vi "Sequence.SerialsFglb.vi"(7 "Action (get)":T6=enum."get", 8 "error in":errorcluster, 9 "Printed serials in":i32[](array[numeric]), 10 "Serial data in":T4, 11 "Counters in":T3) -> (0 "error out":errorcluster, 1 "Printed serials out":i32[](array[numeric]), 2 "Serial out":i32, 3 "Counters out":T3, 5 "StatusFlags":T2)   [LabVIEW 2016]
uses:
  Sequence.SerialsFglb.Action.ctl
  Sequence.SerialsFglb.SerialData.ctl
  Station/Station.ProductSlot.ctl
  Sequence.Counters.ctl
  Sequence.SerialsFglb.StatusFlags.ctl
  Sequence.SerialsFglb.Data.ctl
  Global/ApplicationGlobal.vi
panel:
  out "Serials":T1[](array[typedef])
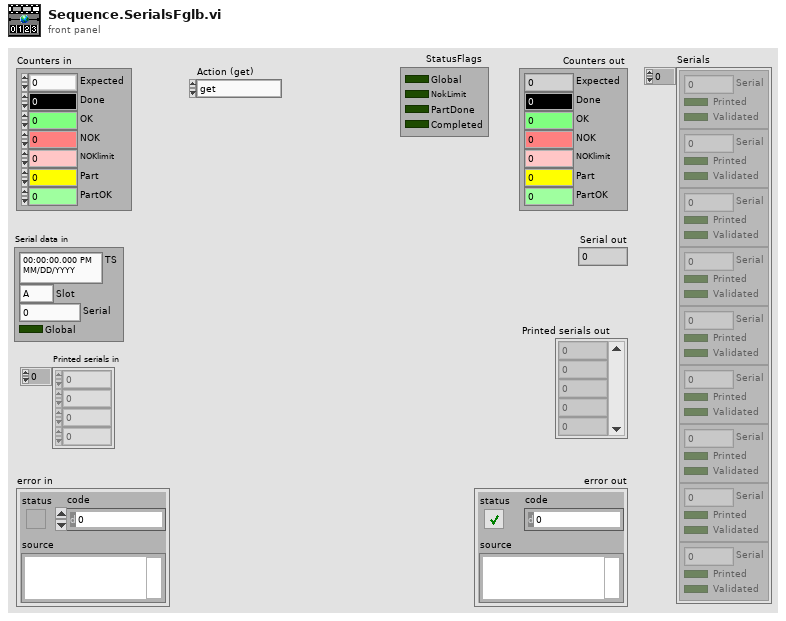
[diagram p1: front panel]
types:
  T1 = typedef "Sequence.SerialsFglb.Data.ctl" = cluster{"Serial":i32, "Printed":bool, "Validated":bool}
  T2 = typedef "Sequence.SerialsFglb.StatusFlags.ctl" = cluster{"Global":bool, "NokLimit":bool, "PartDone":bool, "Completed":bool}
  T3 = typedef "Sequence.Counters.ctl" = cluster{"Expected":u16, "Done":u16, "OK":u16, "NOK":u16, "NOKlimit":u16, "Part":u16, "PartOK":u16}
  T4 = typedef "Sequence.SerialsFglb.SerialData.ctl" = cluster{"TS":timestamp, "Slot":T5, "Serial":i32, "Global":bool}
  T5 = typedef "Station.ProductSlot.ctl" = enum8{"A", "B"}
  T6 = typedef "Sequence.SerialsFglb.Action.ctl" = enum16{"init", "get", "get next", "pass", "fail", "confirm", "clean"}
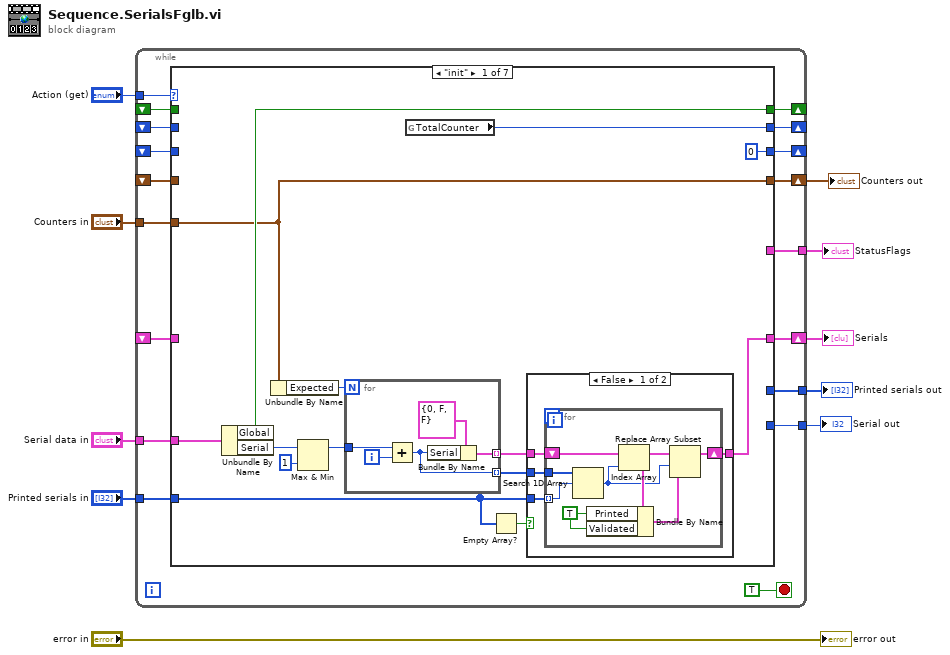
[diagram p0: block diagram]
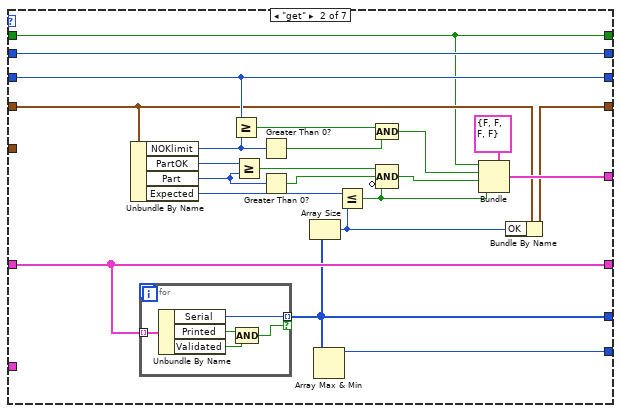
[diagram p3: hidden frame]
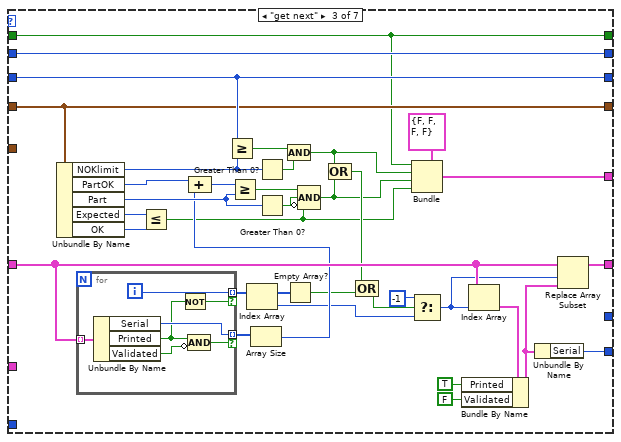
[diagram p4: hidden frame]
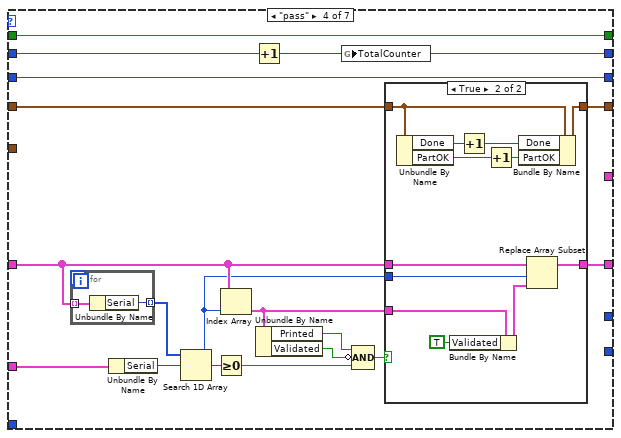
[diagram p5: hidden frame]
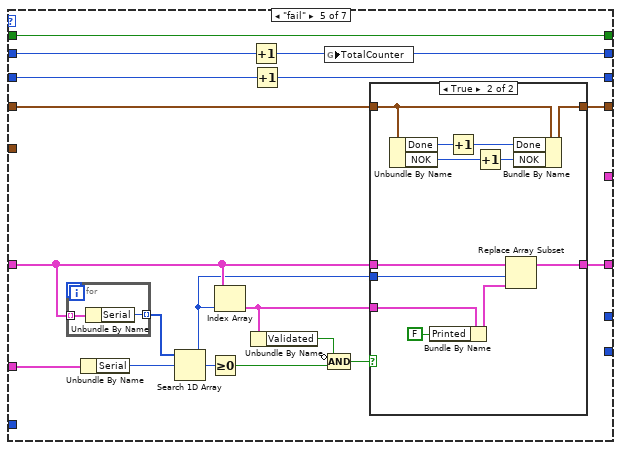
[diagram p7: hidden frame]
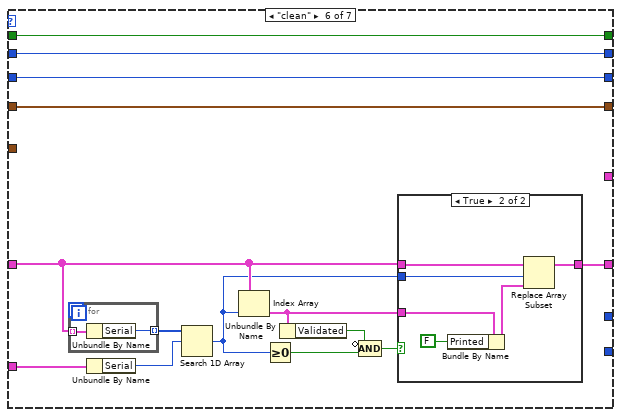
[diagram p9: hidden frame]
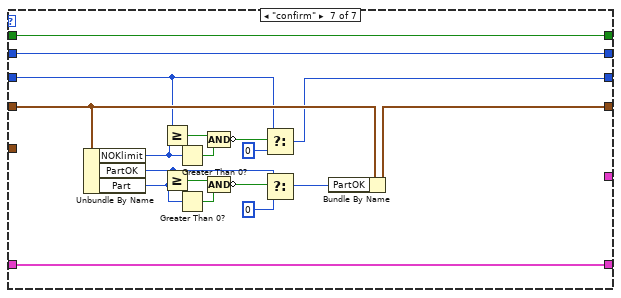
[diagram p11: hidden frame]
diagram:
  n1 = while {
    tunnel: "Action (get)" -> [w27]
    shift-right: [w26] -> w1
    shift-left: _ -> [w25]
    tunnel: [w24] -> w8
    tunnel: "Serial data in" -> [w23]
    tunnel: "Printed serials in" -> [w22]
    tunnel: [w21] -> w5
    shift-right: [w20] -> _
    shift-left: _ -> [w19]
    shift-right: [w17] -> w3
    shift-left: _ -> [w18]
    tunnel: "Counters in" -> [w16]
    shift-right: [w15] -> _
    shift-left: _ -> [w14]
    shift-right: [w13] -> _
    shift-left: _ -> [w12]
    tunnel: [w11] -> w2
    stop <- TRUE stop-if-true
    n2 = case shown="\"init\"" w27 {
      tunnel: [w34 w82 w122 w136 w179 w209 w221] -> w26
      tunnel: w25 -> [_ w82 w121 w137 w169 w208 w221]
      tunnel: [_ w81 w88 _ _ _ _] -> w24
      tunnel: w23 -> [w42 _ _ w145 w165 w207 _]
      tunnel: w22 -> [w37 _ _ _ _ _ _]
      tunnel: [_ w68 _ _ _ _ _] -> w21
      tunnel: [w33 w66 w97 w144 w178 w206 w220] -> w20
      tunnel: w19 -> [_ w66 w97 w144 w178 w206 w220]
      tunnel: w18 -> [_ w70 w106 w140 w174 w203 w226]
      tunnel: [w32 w69 w106 w143 w173 w203 w225] -> w17
      tunnel: w16 -> [w32 _ _ _ _ _ _]
      tunnel: [w29 w80 w117 w139 w172 w205 w222] -> w15
      tunnel: w14 -> [_ w80 w117 w142 w177 w205 w222]
      tunnel: [0 w74 w111 w141 w176 w204 w219] -> w13
      tunnel: w12 -> [_ w74 w111 w141 w175 w204 w223]
      tunnel: [_ w71 w108 _ _ _ _] -> w11
      frame "init" {
        n3 = Unbundle By Name(w42) -> ("Global"=w33:bool, "Serial"=w41:i32)
        n4 = Unbundle By Name(w32) -> ("Expected"=w31:u16)
        n5 = Max & Min(x=w41, y=1) -> (max(x,y)=w35:i32)  [unwired: 1 out]
        n6 = for {
          N: w31 -> [_]
          tunnel: w35 -> [w60]
          tunnel: [w57] -> w39 mode=indexing
          tunnel: [w56] -> w38 mode=indexing
          i -> [w59]
          n7 = Add(x=w60, y=w59) -> (x+y=w56:i32)
          n8 = Bundle By Name(cluster=T1 {"Serial"=0, "Printed"=FALSE, "Validated"=FALSE} ("Data"), "Serial"=w56) -> (w57:T1)
        }
        n9 = global read "ApplicationGlobal.vi" "TotalCounter"() -> (w29:u32)
        n10 = Empty Array?(array=w37) -> (empty?=w36:bool)
        n11 = case shown="False" w36 {
          tunnel: w39 -> [w46 w55]
          tunnel: w38 -> [w45 _]
          tunnel: w37 -> [w44 _]
          tunnel: [w43 w55] -> w34
          frame False {
            n12 = for {
              tunnel: w45 -> [w54]
              tunnel: w44 -> [w53] mode=indexing
              shift-right: [w52] -> w43
              shift-left: w46 -> [w51]
              w49 = TRUE ("Printed")
              n13 = Search 1D Array(1D array=w54, element=w53) -> (index of element=w47:i32)  [unwired: 1 in]
              n14 = Index Array(array=w51, index=w47) -> (element=w50:T1)
              n15 = Bundle By Name(cluster=w50, "Printed"=w49, "Validated"=w49) -> (w48:T1)
              n16 = Replace Array Subset(array=w51, new element=w48, index=w47) -> (w52:T1[])
            }
          }
          frame True {
          }
        }
      }
      frame "get" {
        n17 = Unbundle By Name(w70) -> ("NOKlimit"=w73:u16, "PartOK"=w75:u16, "Part"=w76:u16, "Expected"=w67:u16)
        n18 = for {
          tunnel: w82 -> [w87] mode=indexing
          tunnel: [w86] -> w68 mode=indexing if=w83
          n19 = Unbundle By Name(w87) -> ("Serial"=w86:i32, "Printed"=w85:bool, "Validated"=w84:bool)
          n20 = Compound Arithmetic op=AND(w85, w84) -> (w83:bool)
        }
        n21 = Greater Or Equal?(x=w74, y=w73) -> (x >= y?=w79:bool)
        n22 = Greater Or Equal?(x=w75, y=w76) -> (x >= y?=w77:bool)
        n23 = Greater Than 0?(x=w73) -> (x > 0?=w78:bool)
        n24 = Greater Than 0?(x=w76) -> (x > 0?=w62:bool)
        n25 = Array Size(array=w68) -> (size(s)=w63:i32)
        n26 = Array Max & Min(array=w68) -> (max value=w81:i32)  [unwired: 3 out]
        n27 = Less Or Equal?(x=w67, y=w63) -> (x <= y?=w61:bool)
        n28 = Compound Arithmetic op=AND(w79, w78) -> (w65:bool)
        n29 = Compound Arithmetic op=AND(w77, w62, invert w61) -> (w64:bool)
        n30 = Bundle(cluster=T2 {"Global"=FALSE, "NokLimit"=FALSE, "PartDone"=FALSE, "Completed"=FALSE} ("StatusFlags"), "Global"=w66, "NokLimit"=w65, "PartDone"=w64, "Completed"=w61) -> (w71:T2)
        n31 = Bundle By Name(cluster=w70, "OK"=w63) -> (w69:T3)
      }
      frame "get next" {
        n32 = Unbundle By Name(w106) -> ("NOKlimit"=w112:u16, "PartOK"=w104:u16, "Part"=w113:u16, "Expected"=w94:u16, "OK"=w93:u16)
        n33 = for {
          tunnel: w121 -> [w129] mode=indexing
          tunnel: [w128] -> w101 mode=indexing if=w127
          tunnel: [w126] -> w105 mode=indexing if=w124
          i -> [w128]
          n34 = Unbundle By Name(w129) -> ("Serial"=w126:i32, "Printed"=w125:bool, "Validated"=w123:bool)
          n35 = Not(x=w125) -> (.not. x?=w127:bool)
          n36 = Compound Arithmetic op=AND(w125, invert w123) -> (w124:bool)
        }
        n37 = Less Or Equal?(x=w94, y=w93) -> (x <= y?=w91:bool)
        n38 = Greater Or Equal?(x=w111, y=w112) -> (x >= y?=w116:bool)
        n39 = Index Array(array=w101) -> (element=w98:i32)  [unwired: 1 in]
        n40 = Array Size(array=w105) -> (size(s)=w102:i32)
        n41 = Compound Arithmetic op=ADD(w104, w102) -> (w103:i32)
        n42 = Greater Or Equal?(x=w103, y=w113) -> (x >= y?=w114:bool)
        n43 = Greater Than 0?(x=w112) -> (x > 0?=w115:bool)
        n44 = Greater Than 0?(x=w113) -> (x > 0?=w92:bool)
        n45 = Empty Array?(array=w101) -> (empty?=w100:bool)
        n46 = Compound Arithmetic op=AND(w116, w115) -> (w96:bool)
        n47 = Compound Arithmetic op=AND(w114, w92, invert w91) -> (w95:bool)
        n48 = Compound Arithmetic op=OR(w96, w95) -> (w110:bool)
        n49 = Compound Arithmetic op=OR(w110, w100) -> (w107:bool)
        n50 = Bundle(cluster=T2 {"Global"=FALSE, "NokLimit"=FALSE, "PartDone"=FALSE, "Completed"=FALSE} ("StatusFlags"), "Global"=w97, "NokLimit"=w96, "PartDone"=w95, "Completed"=w91) -> (w108:T2)
        n51 = Select(t=-1 ("f"), s=w107, f=w98) -> (s? t:f=w120:i32)
        n52 = Index Array(array=w121, index=w120) -> (element=w119:T1)
        n53 = Bundle By Name(cluster=w119, "Printed"=TRUE, "Validated"=FALSE) -> (w89:T1)
        n54 = Unbundle By Name(w89) -> ("Serial"=w88:i32)
        n55 = Replace Array Subset(array=w121, new element=w89, index=w120) -> (w122:T1[])
      }
      frame "pass" {
        n56 = for {
          tunnel: w137 -> [w148] mode=indexing
          tunnel: [w147] -> w146 mode=indexing
          n57 = Unbundle By Name(w148) -> ("Serial"=w147:i32)
        }
        n58 = Unbundle By Name(w145) -> ("Serial"=w132:i32)
        n59 = Search 1D Array(1D array=w146, element=w132) -> (index of element=w134:i32)  [unwired: 1 in]
        n60 = Greater Or Equal To 0?(x=w134) -> (x >= 0?=w133:bool)
        n61 = Index Array(array=w137, index=w134) -> (element=w135:T1)
        n62 = Increment(x=w142) -> (x+1=w139:u32)
        n63 = Unbundle By Name(w135) -> ("Printed"=w130:bool, "Validated"=w131:bool)
        n64 = global write "ApplicationGlobal.vi" "TotalCounter"(w139) -> ()
        n65 = Compound Arithmetic op=AND(w130, invert w131, w133) -> (w138:bool)
        n66 = case shown="True" w138 {
          tunnel: w140 -> [w150 w162]
          tunnel: [w150 w161] -> w143
          tunnel: w137 -> [w149 w156]
          tunnel: [w149 w155] -> w136
          tunnel: w135 -> [_ w154]
          tunnel: w134 -> [_ w153]
          frame False {
          }
          frame True {
            n67 = Unbundle By Name(w162) -> ("Done"=w152:u16, "PartOK"=w160:u16)
            n68 = Bundle By Name(cluster=w154, "Validated"=TRUE ("Printed")) -> (w158:T1)
            n69 = Increment(x=w152) -> (x+1=w151:u16)
            n70 = Increment(x=w160) -> (x+1=w159:u16)
            n71 = Bundle By Name(cluster=w162, "Done"=w151, "PartOK"=w159) -> (w161:T3)
            n72 = Replace Array Subset(array=w156, new element=w158, index=w153) -> (w155:T1[])
          }
        }
      }
      frame "fail" {
        n73 = for {
          tunnel: w169 -> [w195] mode=indexing
          tunnel: [w194] -> w171 mode=indexing
          n74 = Unbundle By Name(w195) -> ("Serial"=w194:i32)
        }
        n75 = Unbundle By Name(w165) -> ("Serial"=w164:i32)
        n76 = Search 1D Array(1D array=w171, element=w164) -> (index of element=w166:i32)  [unwired: 1 in]
        n77 = Greater Or Equal To 0?(x=w166) -> (x >= 0?=w170:bool)
        n78 = Index Array(array=w169, index=w166) -> (element=w168:T1)
        n79 = Increment(x=w177) -> (x+1=w172:u32)
        n80 = Unbundle By Name(w168) -> ("Validated"=w163:bool)
        n81 = Increment(x=w175) -> (x+1=w176:i32)
        n82 = global write "ApplicationGlobal.vi" "TotalCounter"(w172) -> ()
        n83 = Compound Arithmetic op=AND(invert w163, w170) -> (w167:bool)
        n84 = case shown="True" w167 {
          tunnel: [w180 w193] -> w179
          tunnel: w174 -> [w181 w189]
          tunnel: [w181 w186] -> w173
          tunnel: w169 -> [w180 w184]
          tunnel: w168 -> [_ w183]
          tunnel: w166 -> [_ w182]
          frame False {
          }
          frame True {
            n85 = Unbundle By Name(w189) -> ("Done"=w190:u16, "NOK"=w188:u16)
            n86 = Bundle By Name(cluster=w183, "Printed"=FALSE) -> (w192:T1)
            n87 = Increment(x=w190) -> (x+1=w191:u16)
            n88 = Increment(x=w188) -> (x+1=w187:u16)
            n89 = Replace Array Subset(array=w184, new element=w192, index=w182) -> (w193:T1[])
            n90 = Bundle By Name(cluster=w189, "Done"=w191, "NOK"=w187) -> (w186:T3)
          }
        }
      }
      frame "clean" {
        n91 = for {
          tunnel: w208 -> [w218] mode=indexing
          tunnel: [w217] -> w202 mode=indexing
          n92 = Unbundle By Name(w218) -> ("Serial"=w217:i32)
        }
        n93 = Unbundle By Name(w207) -> ("Serial"=w200:i32)
        n94 = Search 1D Array(1D array=w202, element=w200) -> (index of element=w201:i32)  [unwired: 1 in]
        n95 = Index Array(array=w208, index=w201) -> (element=w199:T1)
        n96 = Greater Or Equal To 0?(x=w201) -> (x >= 0?=w198:bool)
        n97 = Unbundle By Name(w199) -> ("Validated"=w196:bool)
        n98 = Compound Arithmetic op=AND(invert w196, w198) -> (w197:bool)
        n99 = case shown="True" w197 {
          tunnel: [w210 w216] -> w209
          tunnel: w201 -> [_ w214]
          tunnel: w208 -> [w210 w213]
          tunnel: w199 -> [_ w211]
          frame False {
          }
          frame True {
            n100 = Bundle By Name(cluster=w211, "Printed"=FALSE) -> (w215:T1)
            n101 = Replace Array Subset(array=w213, new element=w215, index=w214) -> (w216:T1[])
          }
        }
      }
      frame "confirm" {
        n102 = Unbundle By Name(w226) -> ("NOKlimit"=w224:u16, "PartOK"=w227:u16, "Part"=w231:u16)
        n103 = Greater Or Equal?(x=w223, y=w224) -> (x >= y?=w237:bool)
        n104 = Greater Or Equal?(x=w227, y=w231) -> (x >= y?=w233:bool)
        n105 = Greater Than 0?(x=w224) -> (x > 0?=w236:bool)
        n106 = Greater Than 0?(x=w231) -> (x > 0?=w232:bool)
        n107 = Compound Arithmetic op=AND(w237, w236) -> (invert w235:bool)
        n108 = Compound Arithmetic op=AND(w233, w232) -> (invert w229:bool)
        n109 = Select(t=w223, s=w235, f=0 ("Total")) -> (s? t:f=w219:i32)
        n110 = Select(t=w227, s=w229, f=u16 0 ("Total")) -> (s? t:f=w228:u16)
        n111 = Bundle By Name(cluster=w226, "PartOK"=w228) -> (w225:T3)
      }
    }
  }
  "Serial out" <- w8
  "Printed serials out" <- w5
  "Counters out" <- w3
  "StatusFlags" <- w2
  "Serials" <- w1
  "error out" <- "error in"
